vi "rad_Input App Image Properties Dialog.vi"(8 "error in (no error)":errorcluster, 9 "New Image?":bool, 11 "AppImage Properties":T1) -> (0 "error out":errorcluster, 3 "AppImage Properties":T1, 4 "Cancelled":bool)   [LabVIEW 2016]
uses:
  TypeDefs/rad_Application Image Properties.ctl
  TypeDefs/rad_FPGA Properties.ctl
  TypeDefs/rad_FPGA Flash Properties.ctl
  Util/FP Control/FP Control Functions.ctl
panel:
  in  "Configure Blacklists":bool
  in  "Configure FPGA Flash":bool
  out "Old Version":string
  in  "Description":string
  in  "New Version":string
  in  "Name":string
  in  "Cancel Button":bool
  in  "OK Button":bool
  # "Application Image Properties"
  # "Old Version"
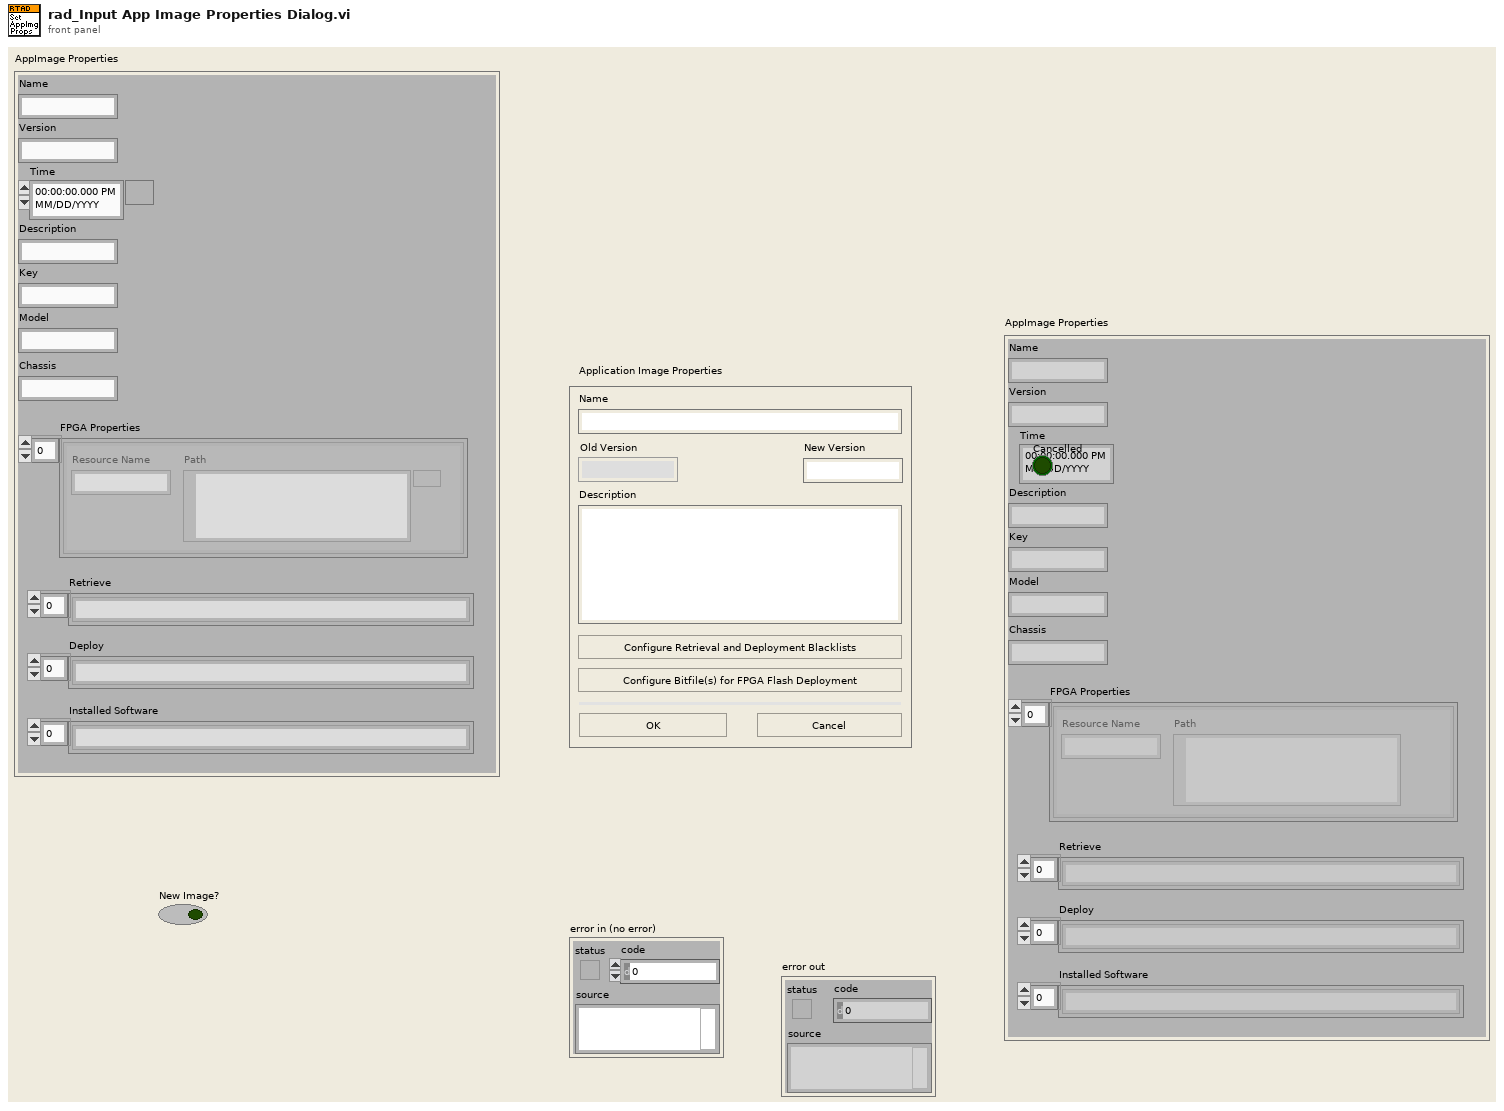
[diagram p1: front panel]
types:
  T1 = typedef "rad_Application Image Properties.ctl" = cluster{"Name":string, "Version":string, "Time":timestamp, "Description":string, "Key":string, "Chassis":string, "FPGA Properties":T2, "Model":string, "Retrieve":string[], "Deploy":string[], "Installed Software":string[]}
  T2 = typedef "rad_FPGA Properties.ctl" = T3[]
  T3 = typedef "rad_FPGA Flash Properties.ctl" = cluster{"Resource Name":string, "Path":path}
  T4 = typedef "FP Control Functions.ctl" = enum16{"Open", "Close", "Bring To Front", "Center"}
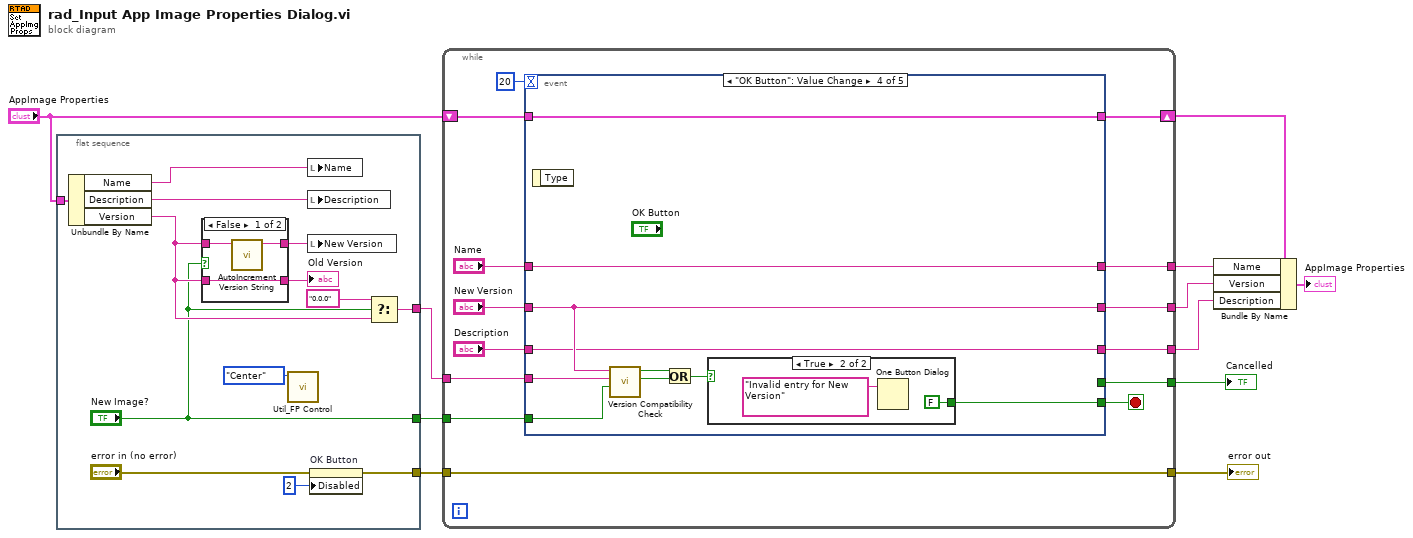
[diagram p0: block diagram]
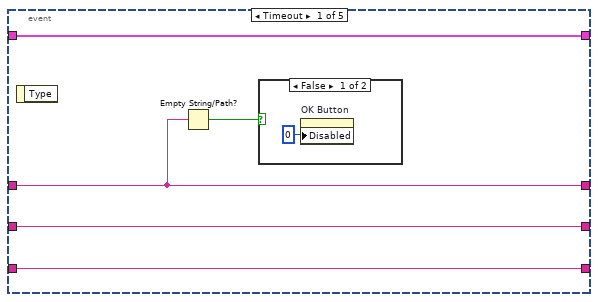
[diagram p3: hidden frame]
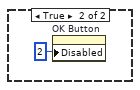
[diagram p4: hidden frame]
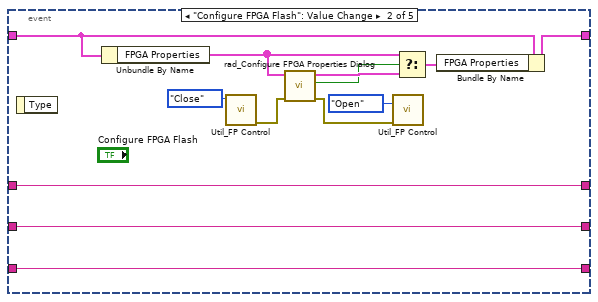
[diagram p5: hidden frame]
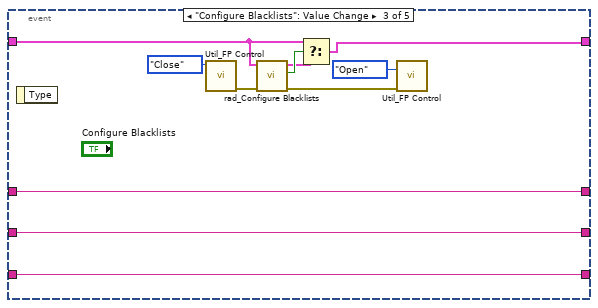
[diagram p6: hidden frame]
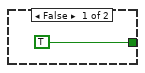
[diagram p7: hidden frame]
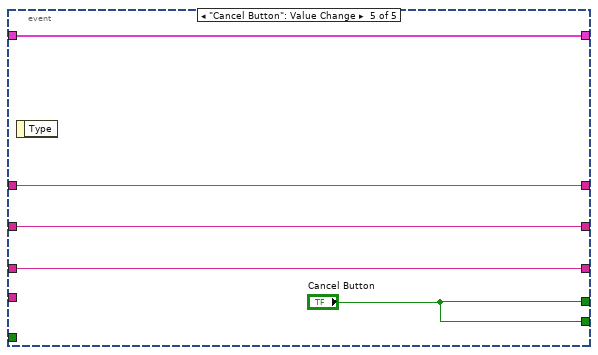
[diagram p8: hidden frame]
diagram:
  n1 = flat-sequence {
    tunnel: [w15] -> w11
    tunnel: "AppImage Properties" -> [w24]
    tunnel: [w16] -> w5
    tunnel: ["New Image?"] -> w4
    frame #0 {
      n2 = Unbundle By Name(w24) -> ("Name"=w13:string, "Description"=w12:string, "Version"=w19:string)
      n3 = case shown="False" "New Image?" {
        tunnel: [w25 w28] -> w21
        tunnel: w19 -> [w27 w28]
        tunnel: w19 -> [w26 _]
        tunnel: [w26 _] -> w23
        frame False {
          n4 = call "AutoIncrement Version String.vi"("Version String"=w27) -> ("AutoIncrement String"=w25:string)  [unwired: 9 in, 1 out]
        }
        frame True {
        }
      }
      "Old Version" <- w23
      n5 = call "Util_FP Control.vi"("Function"=FP_Control_Functions."Center") -> ()  [unwired: 1 in, 10 out]
      n6 = local write "Name"(w13) -> ()
      n7 = local write "Description"(w12) -> ()
      n8 = local write "New Version"(w21) -> ()
      n9 = property on="OK Button" class="Bool"(error in="error in (no error)", "Disabled"=2) -> (error out=w15:errorcluster)  [unwired: 1 in, 1 out]
      n10 = Select(t="0.0.0", s="New Image?", f=w19) -> (s? t:f=w16:string)
    }
  }
  n11 = while {
    tunnel: [w38] -> w8
    tunnel: [w39] -> w7
    tunnel: [w29] -> w9
    tunnel: [w42] -> w10
    tunnel: w11 -> [w42]
    tunnel: w5 -> [w36]
    tunnel: w4 -> [w35]
    tunnel: [w33] -> w1
    shift-right: [w31] -> w2
    shift-left: "AppImage Properties" -> [w32]
    stop <- w34 stop-if-true
    n12 = event shown="[3] \"OK Button\": Value Change" {
      selector: _ -> [_ _ _ _ _]
      dyn-events: _ -> [_ _ _ _ _]
      timeout: 20 -> [_ _ _ _ _]
      tunnel: "Name" -> [w44 w52 w71 w76 w89]
      tunnel: "Description" -> [w45 w50 w69 w74 w87]
      tunnel: [w44 w52 w71 w76 w89] -> w29
      tunnel: [w46 w51 w70 w75 w88] -> w39
      tunnel: [w45 w50 w69 w74 w87] -> w38
      tunnel: "New Version" -> [w46 w51 w70 w75 w88]
      tunnel: w36 -> [_ _ _ w80 _]
      tunnel: w35 -> [_ _ _ w79 _]
      tunnel: [_ _ _ w78 "Cancel Button"] -> w34
      tunnel: [_ _ _ _ "Cancel Button"] -> w33
      tunnel: w32 -> [w47 w62 w63 w77 w90]
      tunnel: [w47 w61 w64 w77 w90] -> w31
      event Timeout {
        n13 = event-data() -> ()  [unwired: 1 in, 1 out]
        n14 = Empty String/Path?(string/path=w44) -> (empty?=w43:bool)
        n15 = case shown="False" w43 {
          frame False {
            n16 = property on="OK Button" class="Bool"("Disabled"=u8 0) -> ()  [unwired: 2 in, 2 out]
          }
          frame True {
            n17 = property on="OK Button" class="Bool"("Disabled"=u8 2) -> ()  [unwired: 2 in, 2 out]
          }
        }
      }
      event "Configure FPGA Flash": Value Change {
        n18 = event-data() -> ()  [unwired: 1 in, 1 out]
        n19 = Unbundle By Name(w62) -> ("FPGA Properties"=w54:T2)
        n20 = call "Util_FP Control.vi"("Function"=FP_Control_Functions."Close") -> ("error out"=w59:errorcluster)  [unwired: 1 in, 9 out]
        n21 = call "rad_Configure FPGA Properties Dialog.vi"("error in (no error)"=w59, "FPGA Properties"=w54) -> ("error out"=w58:errorcluster, "Canceled"=w55:bool, "FPGA Properties Out"=w56:T2)  [unwired: 7 in]
        n22 = call "Util_FP Control.vi"("error in (no error)"=w58, "Function"=FP_Control_Functions."Open") -> ()  [unwired: 10 out]
        n23 = Select(t=w54, s=w55, f=w56) -> (s? t:f=w53:T2)
        n24 = Bundle By Name(cluster=w62, "FPGA Properties"=w53) -> (w61:T1)
      }
      event "Configure Blacklists": Value Change {
        n25 = event-data() -> ()  [unwired: 1 in, 1 out]
        n26 = call "Util_FP Control.vi"("Function"=FP_Control_Functions."Close") -> ("error out"=w68:errorcluster)  [unwired: 1 in, 9 out]
        n27 = call "rad_Configure Blacklists.vi"("error in (no error)"=w68, "AppImage Properties In"=w63) -> ("error out"=w67:errorcluster, "Canceled"=w66:bool, "AppImage Properties Out"=w65:T1)  [unwired: 7 in]
        n28 = Select(t=w63, s=w66, f=w65) -> (s? t:f=w64:T1)
        n29 = call "Util_FP Control.vi"("error in (no error)"=w67, "Function"=FP_Control_Functions."Open") -> ()  [unwired: 10 out]
      }
      event "OK Button": Value Change {
        n30 = event-data() -> ()  [unwired: 1 in, 1 out]
        n31 = call "Version Compatibility Check.vi"("Allow Equal?"=w79, "Old Version"=w80, "New Version"=w75) -> ("Incompatible?"=w82:bool, "Invalid Format?"=w83:bool)  [unwired: 7 in]
        n32 = Or(x=w83, y=w82) -> (x .or. y?=w81:bool)
        n33 = case shown="True" w81 {
          tunnel: [TRUE FALSE] -> w78
          frame False {
          }
          frame True {
            n34 = One Button Dialog(message="Invalid entry for New Version") -> ()  [unwired: 1 in, 1 out]
          }
        }
      }
      event "Cancel Button": Value Change {
        n35 = event-data() -> ()  [unwired: 1 in, 1 out]
      }
    }
  }
  "Cancelled" <- w1
  "error out" <- w10
  n36 = Bundle By Name(cluster=w2, "Name"=w9, "Version"=w7, "Description"=w8) -> (→"AppImage Properties":T1)
